vi "BASE_I_O_Screen.vi"(8 "error in (no error)":errorcluster) -> (0 "error out":errorcluster)   [LabVIEW 2017]
doc: "This vi is for manually turn ON and OFF also monitor Output of PLCS. So this is manual screen."
panel:
  out "Y22 2":bool
  out "Y25":bool
  out "Y23":bool
  out "Y22":bool
  out "Y21":bool
  out "Y20-SPARE":bool
  out "X27-SPARE":bool
  out "X26-SPARE":bool
  out "X25-REJECTION FULL SENSOR":bool
  out "X24-REJECTION SENSOR":bool
  out "X23-DOOR 4":bool
  out "X22-DOOR 3":bool
  out "PART CLAMP END RS":bool
  out "UP DOWN CYL END RS":bool
  out "UP DOWN CYL  HM RS":bool
  out "PUSHER END RS":bool
  out "PUSHER HM RS":bool
  out "THREAD LOCKER CYL COMPLETE":bool
  out "SHUTTLE OPEN CHECK SENSOR-X300":bool
  out "SPARE":bool
  out "DOOR 2":bool
  out "DOOR 1":bool
  out "SAFETY SENSOR":bool
  out "GREEN LAMP":bool
  out "PRESSURE SWITCH":bool
  out "RESET PB":bool
  out "EMG STOP":bool
  out "CYCLE START TOUCH BUTTON 2":bool
  out "CYCLE START TOUCH BUTTON 1":bool
  out "BUZZER":bool
  out "RED LAMP":bool
  out "AUTO/MANUAL":bool
  out "UP DN CYL REV SOL":bool
  out "UP DN CYL FWD SOL":bool
  out "PUSHER REV SOL":bool
  out "PUSHER FWD SOL":bool
  out "THREAD LOCKER OFF":bool
  out "THREAD LOCKER ON":bool
  out "PART CLAMP SOL":bool
  in  "Back":bool
  # "BARCODE VERIFICATION SYSTEM REPORTS"
  # "I/O Screen"
  # "INPUT"
  # "OUTPUT"
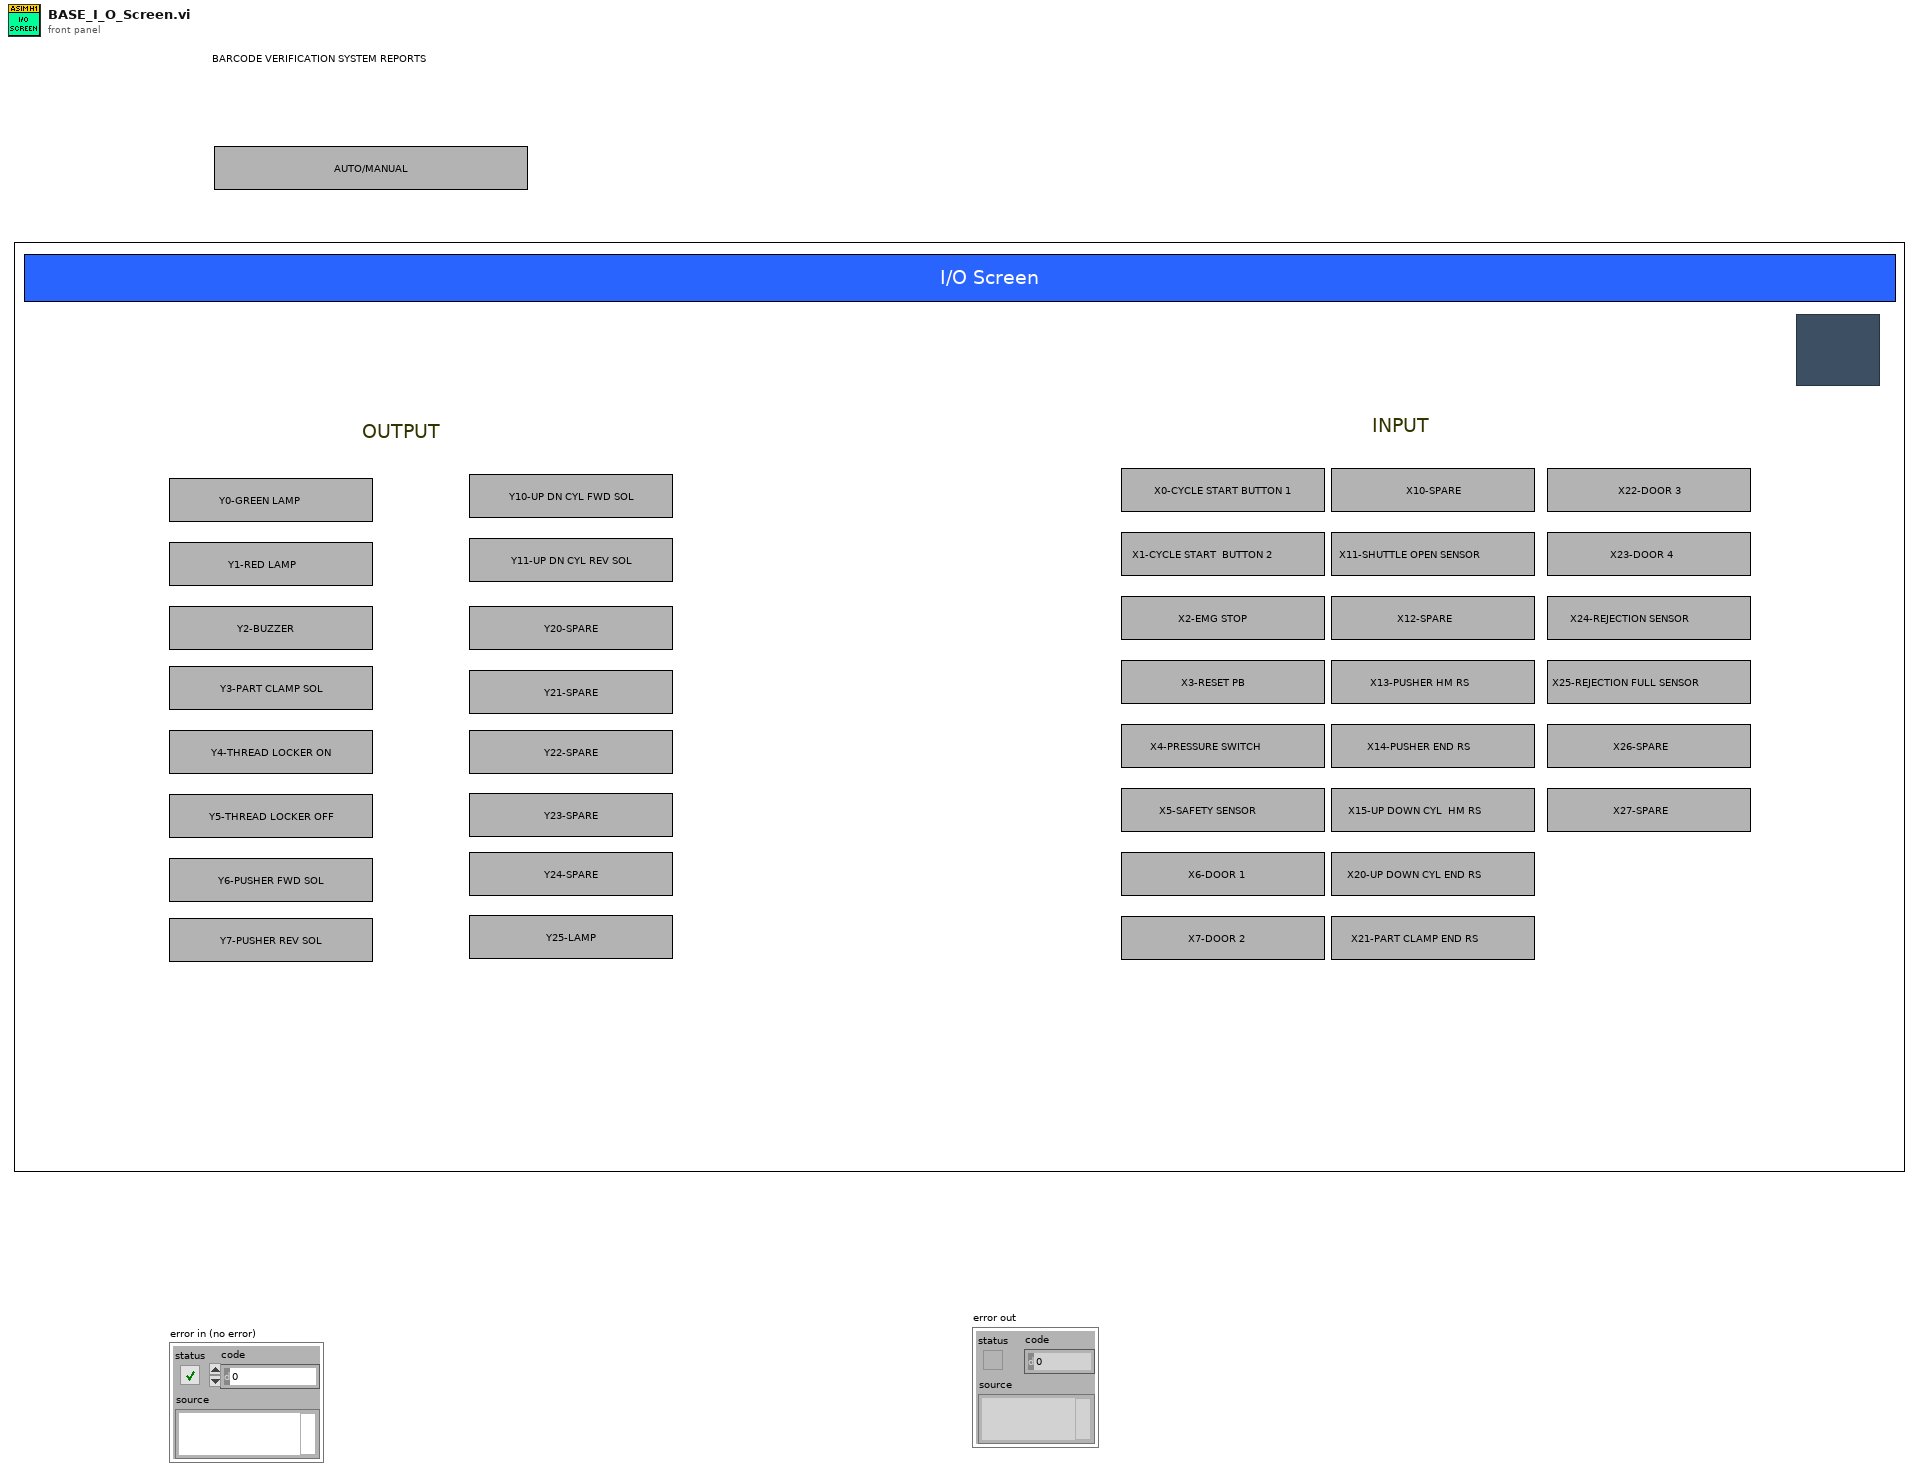
[diagram p1: front panel]
types:
  T1 = enum32{"invalid app kind", "Development System", "Run Time System", "Student Edition", "Embedded LabVIEW", "Evaluation", "Custom"}
  T2 = enum32{"Invalid", "Standard", "Closed", "Hidden", "Minimized", "Maximized"}
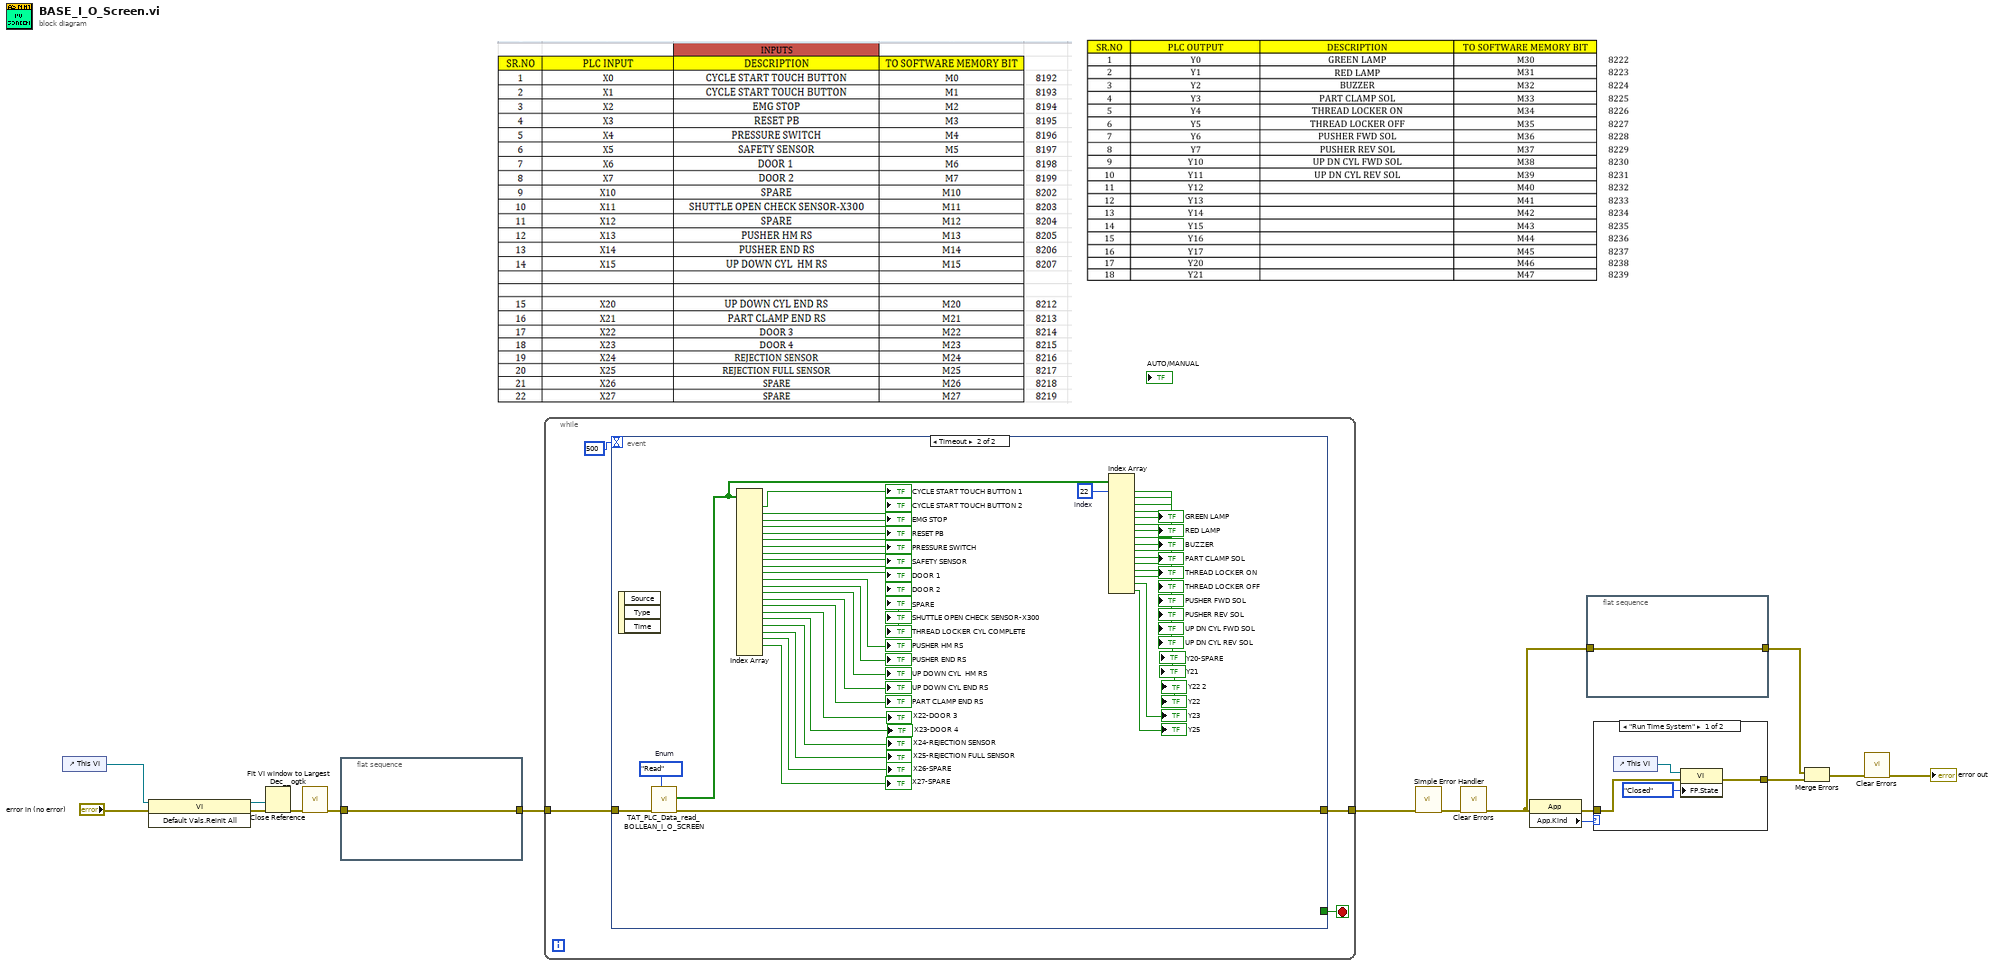
[diagram p0: block diagram]
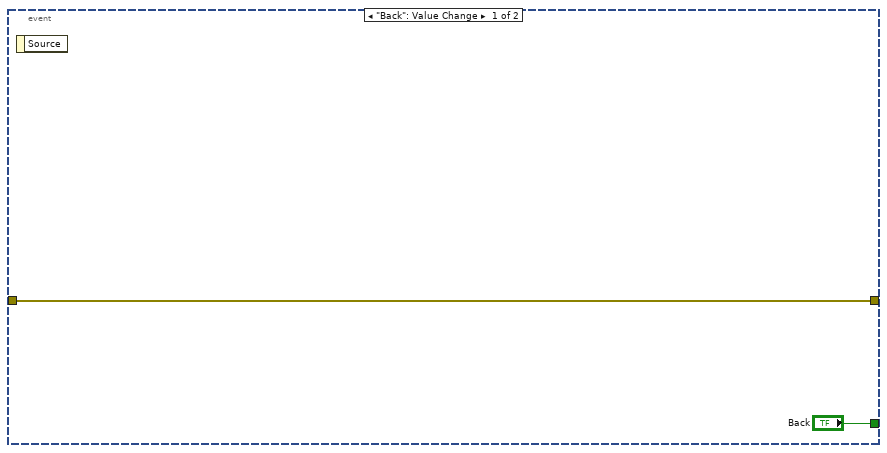
[diagram p3: hidden frame]
diagram:
  n1 = control-ref of="This VI"() -> (w12:refnum<vi>)
  n2 = invoke class="VI" method="Default Vals.Reinit All"(reference=w12, error in="error in (no error)") -> (reference out=w10:refnum<vi>, error out=w9:errorcluster)  [unwired: 1 in, 1 out]
  n3 = Close Reference(reference=w10, error in (no error)=w9) -> (error out=w8:errorcluster)
  n4 = call <userlib>:"Fit VI window to Largest Dec__ogtk.vi"("error in (no error)"=w8) -> ("error out"=w7:errorcluster)  [unwired: 5 in, 1 out]
  n5 = flat-sequence {
    tunnel: w7 -> [w17]
    tunnel: [w17] -> w3
    frame #0 {
    }
  }
  n6 = while {
    tunnel: w3 -> [w21]
    tunnel: [w20] -> w15
    stop <- w19 stop-if-true
    n7 = event shown="[1] Timeout" {
      selector: _ -> [_ _]
      dyn-events: _ -> [_ _]
      timeout: 500 -> [_ _]
      tunnel: w21 -> [w22 w65]
      tunnel: [w22 w64] -> w20
      tunnel: ["Back" _] -> w19
      event "Back": Value Change {
        n8 = event-data() -> ()  [unwired: 1 in, 1 out]
      }
      event Timeout {
        w40 = 22  # index
        w66 = enum16{"Read", "Write"}."Read"  # Enum
        n9 = event-data() -> ()  [unwired: 1 in, 3 out]
        n10 = call "TAT_PLC_Data_read_BOLLEAN_I_O_SCREEN.vi"("Enum"=w66, "error in (no error)"=w65) -> ("error out"=w64:errorcluster, "Array 2"=w41:bool[])  [unwired: 8 in]
        n11 = Index Array(array=w41) -> (element #1=→"CYCLE START TOUCH BUTTON 1":bool, element #2=→"CYCLE START TOUCH BUTTON 2":bool, element #3=→"EMG STOP":bool, element #4=→"RESET PB":bool, element #5=→"PRESSURE SWITCH":bool, element #6=→"SAFETY SENSOR":bool, element #7=→"DOOR 1":bool, element #8=→"DOOR 2":bool, element #9=→"SPARE":bool, element #10=→"SHUTTLE OPEN CHECK SENSOR-X300":bool, element #11=→"THREAD LOCKER CYL COMPLETE":bool, element #12=→"PUSHER HM RS":bool, element #13=→"PUSHER END RS":bool, element #14=→"UP DOWN CYL  HM RS":bool, element #15=→"UP DOWN CYL END RS":bool, element #16=→"PART CLAMP END RS":bool, element #17=→"X22-DOOR 3":bool, element #18=→"X23-DOOR 4":bool, element #19=→"X24-REJECTION SENSOR":bool, element #20=→"X25-REJECTION FULL SENSOR":bool, element #21=→"X26-SPARE":bool, element #22=→"X27-SPARE":bool)  [unwired: 23 in, 1 out]
        n12 = Index Array(array=w41, index #1=w40) -> (element #1=→"GREEN LAMP":bool, element #2=→"RED LAMP":bool, element #3=→"BUZZER":bool, element #4=→"PART CLAMP SOL":bool, element #5=→"THREAD LOCKER ON":bool, element #6=→"THREAD LOCKER OFF":bool, element #7=→"PUSHER FWD SOL":bool, element #8=→"PUSHER REV SOL":bool, element #9=→"UP DN CYL FWD SOL":bool, element #10=→"UP DN CYL REV SOL":bool, element #11=→"Y20-SPARE":bool, element #12=→"Y21":bool, element #13=→"Y22 2":bool, element #14=→"Y22":bool, element #15=→"Y23":bool, element #16=→"Y25":bool)  [unwired: 15 in]
      }
    }
  }
  n13 = call <vilib>:"Simple Error Handler.vi"("error in (no error)"=w15) -> ("error out"=w6:errorcluster)  [unwired: 4 in, 4 out]
  n14 = call <vilib>:"Clear Errors.vi"("error in (no error)"=w6) -> ("error out"=w2:errorcluster)  [unwired: 5 in, 1 out]
  n15 = property class="App"(error in=w2) -> (error out=w4:errorcluster, "App.Kind"=w5:T1)  [unwired: 1 in, 1 out]
  n16 = flat-sequence {
    tunnel: w2 -> [w67]
    tunnel: [w67] -> w1
    frame #0 {
    }
  }
  n17 = case shown="\"Run Time System\"" w5 {
    tunnel: w4 -> [w69 w72]
    tunnel: [w68 w72] -> w13
    frame "Run Time System" {
      n18 = control-ref of="This VI"() -> (w71:refnum<vi>)
      n19 = property class="VI"(reference=w71, error in=w69, "FP.State"=T2."Closed" ("Front Panel Window:State")) -> (error out=w68:errorcluster)  [unwired: 1 out]
    }
    frame "Development System", Default {
    }
  }
  n20 = Merge Errors(w1, w13) -> (w14:errorcluster)
  n21 = call <vilib>:"Clear Errors.vi"("error in (no error)"=w14) -> ("error out"=→"error out":errorcluster)  [unwired: 5 in, 1 out]
